vi "Get Color.vi"(7 "Splitter? (F: Pane)":bool, 9 "Pane Colors":T1, 10 "UI Selections":T2, 11 "Item Index":i32) -> (3 "Color":u32)   [LabVIEW 2018]
uses:
  <resource>/dialog/QuickDrop/plugins/PaneRelief/Typedefs/UI Selections--Cluster.ctl
  <resource>/dialog/QuickDrop/plugins/PaneRelief/Typedefs/Selection Colors--Cluster.ctl
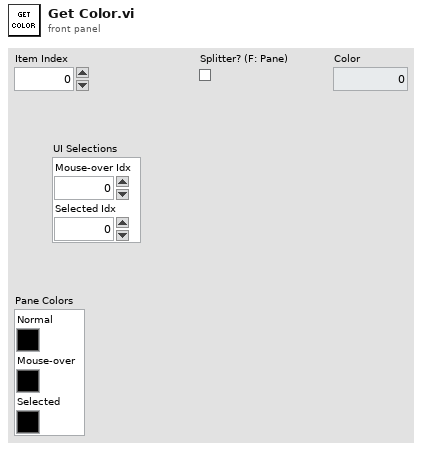
[diagram p1: front panel]
types:
  T1 = typedef "Selection Colors--Cluster.ctl" = cluster{"Normal":u32, "Mouse-over":u32, "Selected":u32}
  T2 = typedef "UI Selections--Cluster.ctl" = cluster{"Mouse-over Idx":i32, "Selected Idx":i32}
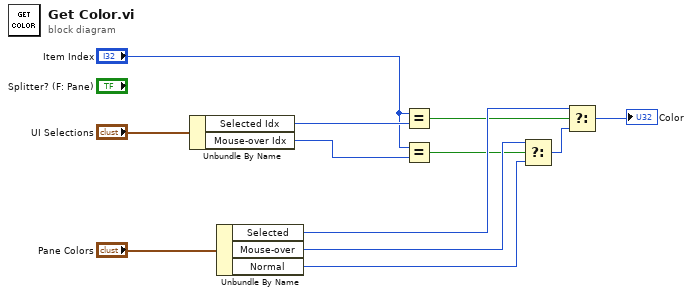
[diagram p0: block diagram]
diagram:
  n1 = Unbundle By Name("UI Selections") -> ("Selected Idx"=w10:i32, "Mouse-over Idx"=w11:i32)
  n2 = Unbundle By Name("Pane Colors") -> ("Selected"=w4:u32, "Mouse-over"=w6:u32, "Normal"=w8:u32)
  n3 = Equal?(x="Item Index", y=w10) -> (x = y?=w2:bool)
  n4 = Equal?(x="Item Index", y=w11) -> (x = y?=w1:bool)
  n5 = Select(t=w6, s=w1, f=w8) -> (s? t:f=w7:u32)
  n6 = Select(t=w4, s=w2, f=w7) -> (s? t:f=→"Color":u32)
